vi "StartJudge.vi"(8 "error in":errorcluster caption="错误输入（无错误）", 9 "CAN通路":T2(ring), 10 "控制簇":T3, 11 "ParaCtl":T1) -> (0 "error out":errorcluster caption="错误输出", 3 "T/F":bool)   [LabVIEW 2013]
uses:
  Ctl/ActionCtl.ctl
  Ctl/ViewCtl.ctl
  USBCAN/DevType.ctl
panel:
  # "ms"
  # "ms"
  # "s"
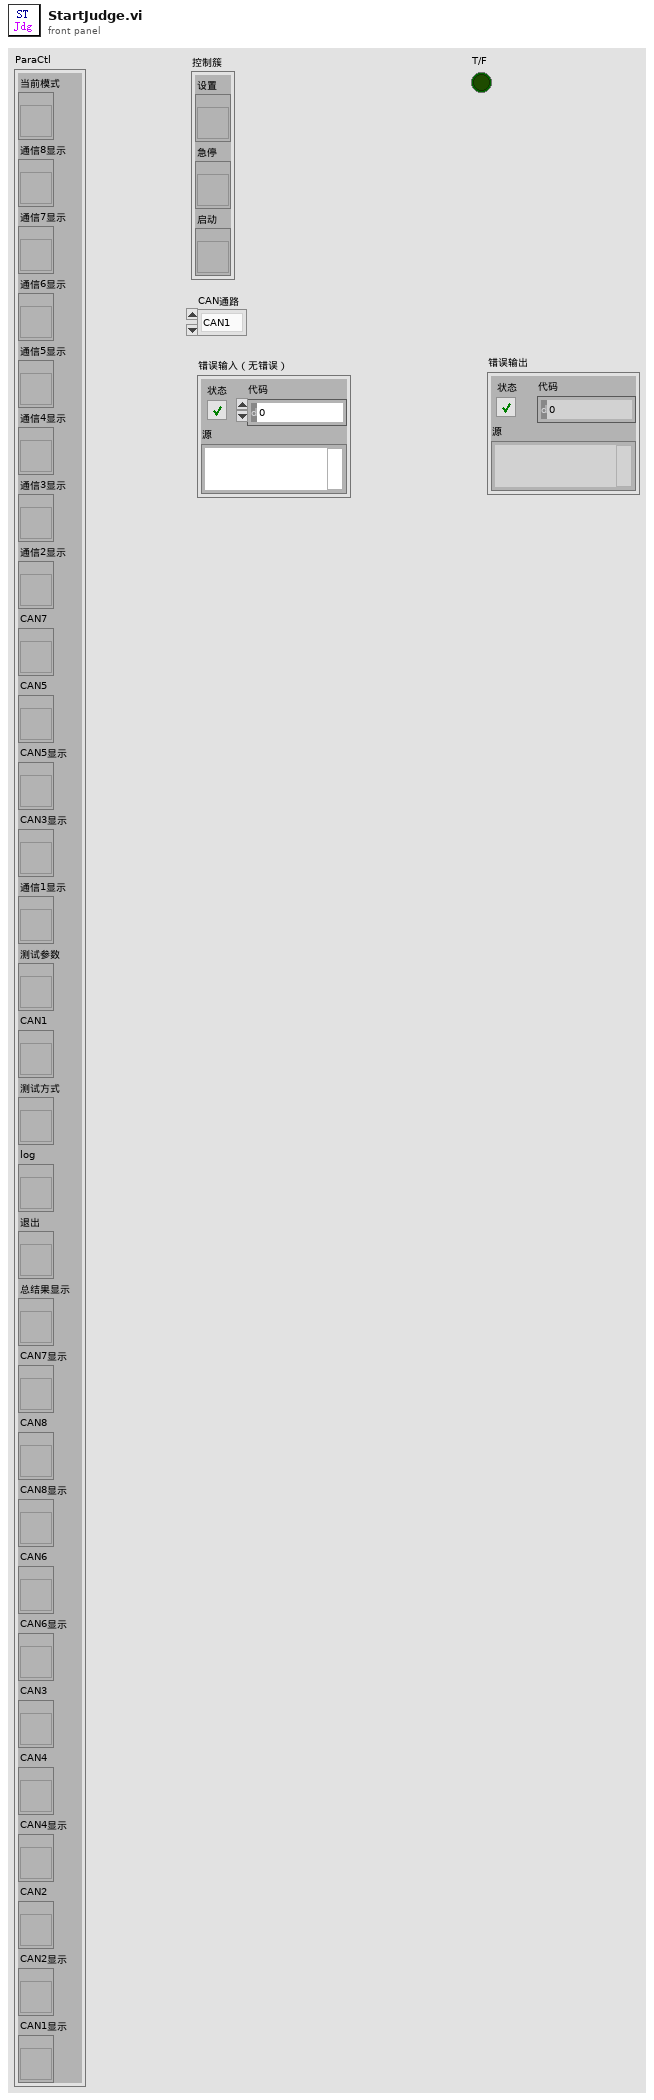
[diagram p1: front panel]
types:
  T1 = typedef "ViewCtl.ctl" = cluster{"当前模式":refnum<vi>, "通信8显示":refnum<vi>, "通信7显示":refnum<vi>, "通信6显示":refnum<vi>, "通信5显示":refnum<vi>, "通信4显示":refnum<vi>, "通信3显示":refnum<vi>, "通信2显示":refnum<vi>, "CAN7":refnum<vi>, "CAN5":refnum<vi>, "CAN5显示":refnum<vi>, "CAN3显示":refnum<vi>, "通信1显示":refnum<vi>, "测试参数":refnum<vi>, "CAN1":refnum<vi>, "测试方式":refnum<vi>, "log":refnum<vi>, "退出":refnum<vi>, "总结果显示":refnum<vi>, "CAN7显示":refnum<vi>, "CAN8":refnum<vi>, "CAN8显示":refnum<vi>, "CAN6":refnum<vi>, "CAN6显示":refnum<vi>, "CAN3":refnum<vi>, "CAN4":refnum<vi>, "CAN4显示":refnum<vi>, "CAN2":refnum<vi>, "CAN2显示":refnum<vi>, "CAN1显示":refnum<vi>}
  T2 = enum16{"CAN1", "CAN2", "CAN3", "CAN4", "CAN5", "CAN6", "CAN7", "CAN8"}
  T3 = typedef "ActionCtl.ctl" = cluster{"设置":refnum<vi>, "急停":refnum<vi>, "启动":refnum<vi>}
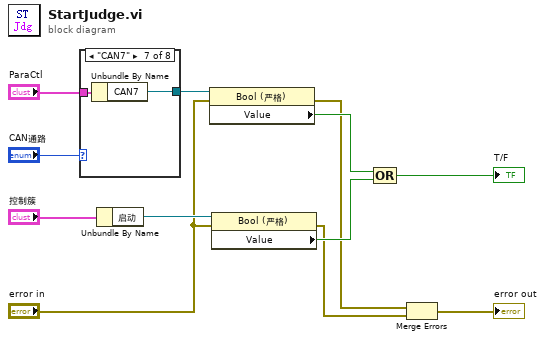
[diagram p0: block diagram]
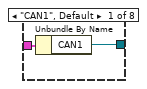
[diagram p2: hidden frame]
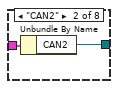
[diagram p3: hidden frame]
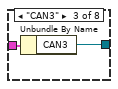
[diagram p4: hidden frame]
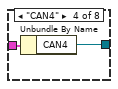
[diagram p5: hidden frame]
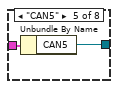
[diagram p6: hidden frame]
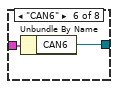
[diagram p7: hidden frame]
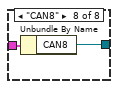
[diagram p8: hidden frame]
diagram:
  n1 = case shown="\"CAN7\"" "CAN通路" {
    tunnel: "ParaCtl" -> [w14 w16 w18 w20 w22 w24 w26 w28]
    tunnel: [w13 w15 w17 w19 w21 w23 w25 w27] -> w12
    frame "CAN1", Default {
      n2 = Unbundle By Name(w14) -> ("CAN1"=w13:refnum<vi>)
    }
    frame "CAN2" {
      n3 = Unbundle By Name(w16) -> ("CAN2"=w15:refnum<vi>)
    }
    frame "CAN3" {
      n4 = Unbundle By Name(w18) -> ("CAN3"=w17:refnum<vi>)
    }
    frame "CAN4" {
      n5 = Unbundle By Name(w20) -> ("CAN4"=w19:refnum<vi>)
    }
    frame "CAN5" {
      n6 = Unbundle By Name(w22) -> ("CAN5"=w21:refnum<vi>)
    }
    frame "CAN6" {
      n7 = Unbundle By Name(w24) -> ("CAN6"=w23:refnum<vi>)
    }
    frame "CAN7" {
      n8 = Unbundle By Name(w26) -> ("CAN7"=w25:refnum<vi>)
    }
    frame "CAN8" {
      n9 = Unbundle By Name(w28) -> ("CAN8"=w27:refnum<vi>)
    }
  }
  n10 = Unbundle By Name("控制簇") -> ("启动"=w10:refnum<vi>)
  n11 = property class="Bool (严格)"(reference=w12, error in="error in") -> (error out=w4:errorcluster, "Value"=w8:bool)  [unwired: 1 out]
  n12 = property class="Bool (严格)"(reference=w10, error in="error in") -> (error out=w3:errorcluster, "Value"=w7:bool)  [unwired: 1 out]
  n13 = Compound Arithmetic op=OR(w8, w7) -> (→"T/F":bool)
  n14 = Merge Errors(w4, w3) -> (→"error out":errorcluster)
